vi "ClientStreamingCancellationTest.vi"() -> (0 "Array of Error Description":T1)   [LabVIEW 2019]
uses:
  gRPC_ATS/TestUtility/utility.llb/array of error description.ctl
  gRPC_ATS/TestUtility/utility.llb/error description.ctl
  gRPC_ATS/TestUtility/utility.llb/error type.ctl
panel:
  out "Pass":bool
  in  "error in (no error)":errorcluster
  in  "Server VI path":path=path "route_guide_server/Run Service.vi"
  in  "Client VI Path":path=path "route_guide_client/ResponseStreaming RouteGuide Test.vi"
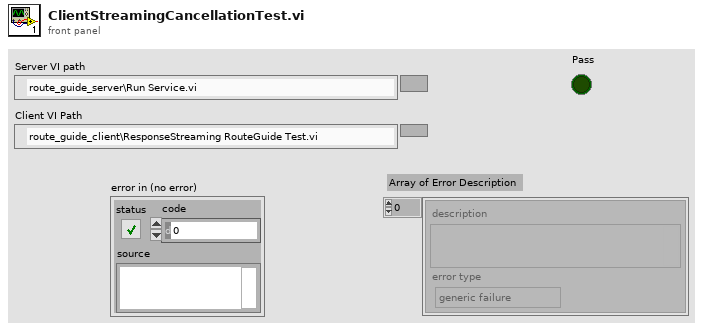
[diagram p1: front panel]
types:
  T1 = typedef "array of error description.ctl" = T2[]
  T2 = typedef "error description.ctl" = cluster{"description":string, "error type":T3}
  T3 = typedef "error type.ctl" = enum32{"generic failure", "boundary case", "precision", "expected error"}
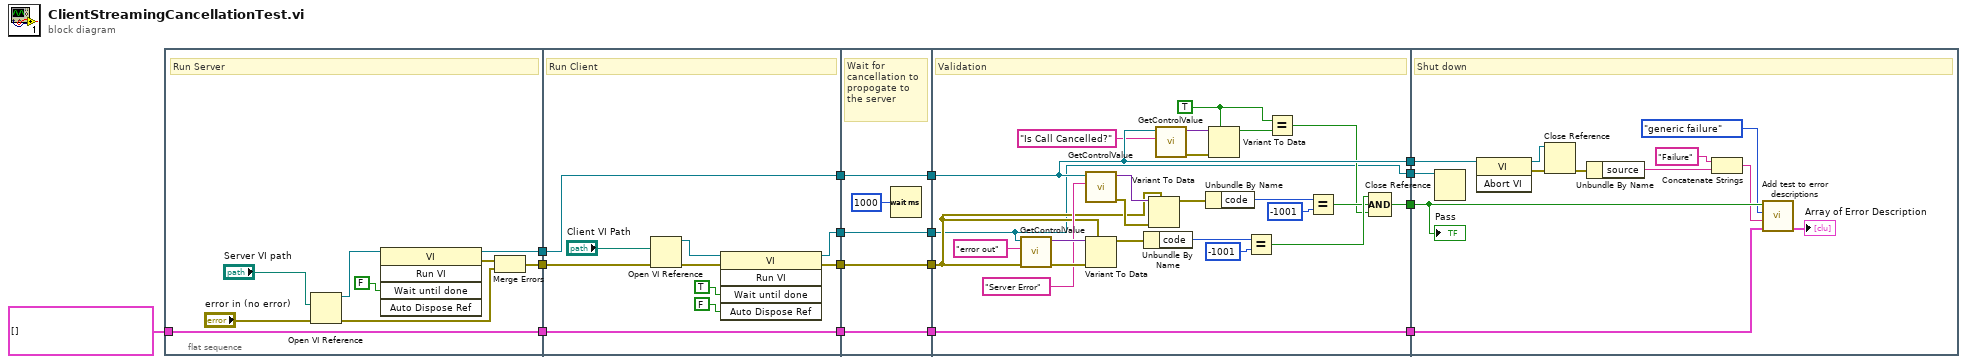
[diagram p0: block diagram]
diagram:
  n1 = flat-sequence {
    tunnel: T1 [] ("error descriptions in") -> [w21]
    tunnel: [w21] -> w14
    tunnel: [w20] -> w11
    tunnel: [w17] -> w10
    tunnel: w14 -> [w34]
    tunnel: [w34] -> w8
    tunnel: [w33] -> w6
    tunnel: w11 -> [w33]
    tunnel: w10 -> [w32]
    tunnel: [w27] -> w4
    tunnel: [w26] -> w2
    tunnel: w8 -> [w40]
    tunnel: [w40] -> w7
    tunnel: w6 -> [w39]
    tunnel: [w39] -> w5
    tunnel: w4 -> [w38]
    tunnel: [w38] -> w3
    tunnel: w2 -> [w37]
    tunnel: [w37] -> w1
    tunnel: [w42] -> w16
    tunnel: w7 -> [w65]
    tunnel: [w65] -> w13
    tunnel: [w58] -> w12
    tunnel: w5 -> [w58]
    tunnel: w3 -> [w41]
    tunnel: w1 -> [w51]
    tunnel: [w41] -> w9
    tunnel: w16 -> [w76]
    tunnel: w13 -> [w71]
    tunnel: w12 -> [w67]
    tunnel: w9 -> [w66]
    frame #0 {
      # "Run Server"
      n2 = Open VI Reference(vi path="Server VI path", error in (no error)="error in (no error)") -> (vi reference=w23:refnum<vi>, error out=w19:errorcluster)  [unwired: 4 in]
      n3 = invoke class="VI" method="Run VI"(reference=w23, "Wait until done"=FALSE ("Wait Until Done")) -> (reference out=w20:refnum<vi>, error out=w18:errorcluster)  [unwired: 3 in, 3 out]
      n4 = Merge Errors(w18, w19) -> (w17:errorcluster)
    }
    frame #1 {
      # "Run Client"
      n5 = Open VI Reference(vi path="Client VI Path", error in (no error)=w32) -> (vi reference=w31:refnum<vi>, error out=w30:errorcluster)  [unwired: 4 in]
      n6 = invoke class="VI" method="Run VI"(reference=w31, error in=w30, "Wait until done"=TRUE ("Wait Until Done"), "Auto Dispose Ref"=FALSE ("Auto Dispose Reference")) -> (reference out=w27:refnum<vi>, error out=w26:errorcluster)  [unwired: 1 in, 3 out]
    }
    frame #2 {
      # "Wait for cancellation to propogate to the server"
      n7 = Wait (ms)(milliseconds to wait=u32 1000) -> ()  [unwired: 1 out]
    }
    frame #3 {
      w46 = TRUE
      # "Validation"
      n8 = call "GetControlValue.vi"("error in (no error)"=w51, "Control Label"="error out", "VI Reference"=w41) -> ("error out"=w62:errorcluster, "Value"=w63:variant)  [unwired: 7 in]
      n9 = call "GetControlValue.vi"("Control Label"="Server Error", "VI Reference"=w58) -> ("error out"=w55:errorcluster, "Value"=w54:variant)  [unwired: 8 in]
      n10 = Variant To Data(error in=w62, type=w51, Variant=w63) -> (data=w61:errorcluster)  [unwired: 1 out]
      n11 = Unbundle By Name(w61) -> ("code"=w60:i32)
      n12 = Variant To Data(error in=w55, type=w51, Variant=w54) -> (data=w48:errorcluster)  [unwired: 1 out]
      n13 = call "GetControlValue.vi"("Control Label"="Is Call Cancelled?", "VI Reference"=w58) -> ("error out"=w53:errorcluster, "Value"=w52:variant)  [unwired: 8 in]
      n14 = Unbundle By Name(w48) -> ("code"=w49:i32)
      n15 = Variant To Data(error in=w53, type=w46, Variant=w52) -> (data=w47:bool)  [unwired: 1 out]
      n16 = Equal?(x=w60, y=-1001) -> (x = y?=w45:bool)
      n17 = Equal?(x=w46, y=w47) -> (x = y?=w43:bool)
      n18 = Equal?(x=w49, y=-1001) -> (x = y?=w44:bool)
      n19 = Compound Arithmetic op=AND(w45, w44, w43) -> (w42:bool)
    }
    frame #4 {
      # "Shut down"
      n20 = Close Reference(reference=w66) -> ()  [unwired: 1 in, 1 out]
      n21 = invoke class="VI" method="Abort VI"(reference=w67) -> (reference out=w69:refnum<vi>, error out=w70:errorcluster)  [unwired: 2 in, 1 out]
      n22 = Close Reference(reference=w69, error in (no error)=w70) -> (error out=w68:errorcluster)
      n23 = Unbundle By Name(w68) -> ("source"=w73:string)
      n24 = Concatenate Strings("Failure" ("string"), w73) -> (w74:string)
      n25 = call "Add test to error descriptions.vi"("error descriptions in"=w71, "error string"=w74, "error type"=error_type."generic failure", "pass"=w76) -> ("error description out"=→"Array of Error Description":T1)  [unwired: 3 in]
      "Pass" <- w76
    }
  }
